vi "GenerateCode.vi"() -> ()   [LabVIEW 2017]
panel:
  in  "RegenerateAll":bool
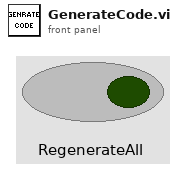
[diagram p1: front panel]
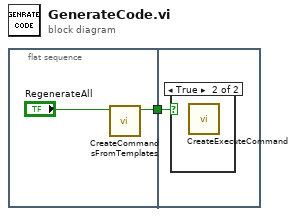
[diagram p0: block diagram]
diagram:
  n1 = flat-sequence {
    tunnel: [w3] -> w1
    tunnel: w1 -> [w4]
    frame #0 {
      n2 = call "CreateCommandsFromTemplates.vi"("RegenerateAll"="RegenerateAll") -> ("NewVI"=w3:bool)  [unwired: 10 in]
    }
    frame #1 {
      n3 = case shown="True" w4 {
        frame False {
        }
        frame True {
          n4 = call "CreateExecuteCommand.vi"() -> ()  [unwired: 12 in]
        }
      }
    }
  }
